vi "Laptop Acquire Image from USB Camera.vi"(8 "Image Name":string, 9 "Y Res":i32, 10 "X Res":i32, 11 "Session In":T1) -> (3 "Image Out":T2(plugin-control))   [LabVIEW 2015]
uses:
  <vilib>/userdefined/High Color/IMAQdx.ctl
  <vilib>/vision/driver/IMAQdx.llb/IMAQdx Camera Control Mode.ctl
  <vilib>/vision/driver/NI_Vision_Acquisition_Software.lvlib
  <vilib>/vision/NI_Vision_Development_Module.lvlib
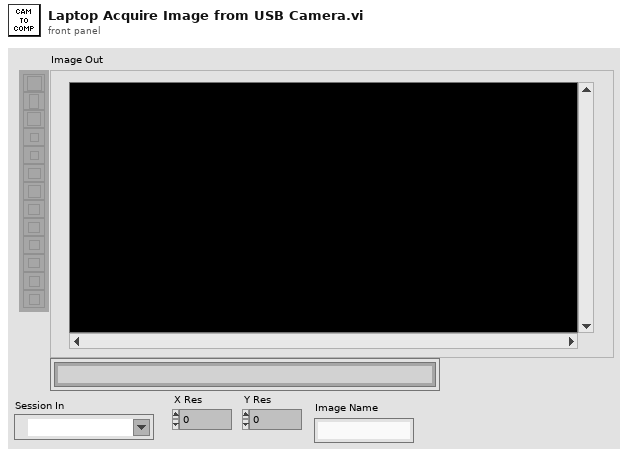
[diagram p1: front panel]
types:
  T1 = typedef "IMAQdx.ctl" = refnum<k21>
  T2 = typedef "IMAQ Image.ctl" = refnum<image>
  T3 = typedef "Image Type" = u32
  T4 = typedef "NI_Vision_Acquisition_Software.lvlib/IMAQdx Camera Control Mode.ctl" = enum32{"Controller", "Listener"}
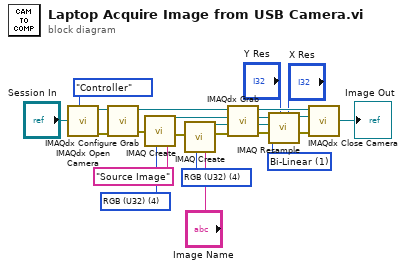
[diagram p0: block diagram]
diagram:
  w2 = u32 1 items=["Zero Order", "Bi-Linear", "Quadratic", "Cubic Spline"] ("Interpolation Type")
  w11 = T3 4 items=["Grayscale (U8)", "Grayscale (I16)", "Grayscale (SGL)", "Complex (CSG)", "RGB (U32)", "HSL (U32)", "RGB (U64)", "Grayscale (U16)"] ("Image Type")
  w14 = T3 4 items=["Grayscale (U8)", "Grayscale (I16)", "Grayscale (SGL)", "Complex (CSG)", "RGB (U32)", "HSL (U32)", "RGB (U64)", "Grayscale (U16)"] ("Image Type")
  n1 = call <vilib>:"IMAQdx Open Camera.vi"("Camera Control Mode"=IMAQdx_Camera_Control_Mode."Controller", "Session In"="Session In") -> ("error out"=w18:errorcluster, "Session Out"=w22:T1)  [unwired: 8 in]
  n2 = call <vilib>:"IMAQdx Configure Grab.vi"("error in"=w18, "Session In"=w22) -> ("error out"=w17:errorcluster, "Session Out"=w21:T1)  [unwired: 8 in]
  n3 = call "IMAQ Create"("Image Name"="Source Image", "Image Type"=w14, "error in (no error)"=w17) -> ("New Image"=w12:T2, "error out"=w9:errorcluster)  [unwired: 2 in]
  n4 = call "IMAQ Create"("Image Name"="Image Name", "Image Type"=w11, "error in (no error)"=w9) -> ("New Image"=w10:T2, "error out"=w8:errorcluster)  [unwired: 2 in]
  n5 = call <vilib>:"IMAQdx Grab.vi"("error in"=w8, "Image In"=w12, "Session In"=w21) -> ("error out"=w1:errorcluster, "Image Out"=w3:T2, "Session Out"=w20:T1)  [unwired: 5 in, 1 out]
  n6 = call "IMAQ Resample"("X Resolution"="X Res", "Y Resolution"="Y Res", "error in (no error)"=w1, "Interpolation Type"=w2, "Image Dst"=w10, "Image Src"=w3) -> ("error out"=w16:errorcluster, "Image Dst Out"=→"Image Out":T2)  [unwired: 4 in]
  n7 = call <vilib>:"IMAQdx Close Camera.vi"("error in"=w16, "Session In"=w20) -> ()  [unwired: 9 in, 1 out]
